vi "SELECT Template.vi"   [LabVIEW 2016]
uses:
  <vilib>/JDP Science/PostgreSQL Library/Result/PQ Result.lvclass
  <vilib>/JDP Science/PostgreSQL Library/Connection/PQ Connection.lvclass
  <vilib>/JDP Science/PostgreSQL Library/Connection/Execute Command (Result).vi
types:
  T1 = cluster{"Get:Get String":string, "Get:Get String":string, "Get:Get String":string, "Get:Get DBL":dbl}
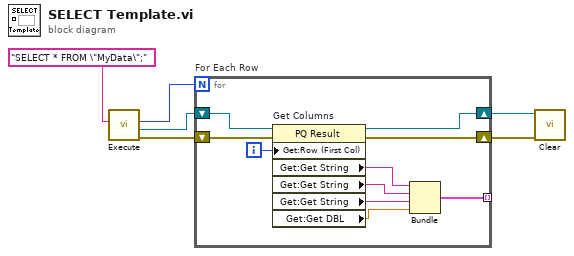
[diagram p0: block diagram]
diagram:
  n1 = call-poly <vilib>:"Execute.vi"("SQL"="SELECT * FROM \"MyData\";" ("command")) -> ("error out"=w4:errorcluster, "First Result with Rows returned"=w1:refnum<class "PQ Result.lvclass">, "Number of Rows"=w5:i32)  [unwired: 7 in, 1 out]
  n2 = for "For Each Row" {
    N: w5 -> [_]
    shift-right: [w16] -> w6
    shift-left: w1 -> [w9]
    shift-right: [w15] -> w3
    shift-left: w4 -> [w8]
    tunnel: [w10] -> _ mode=indexing
    i -> [w7]
    n3 = property on="Get Columns" class="PQ Result"(reference=w9, error in=w8, "Get:Row (First Col)"=w7) -> (reference out=w16:refnum<class "PQ Result.lvclass">, error out=w15:errorcluster, "Get:Get String"=w14:string, "Get:Get String"=w13:string, "Get:Get String"=w12:string, "Get:Get DBL"=w11:dbl)
    n4 = Bundle("Get:Get String"=w14, "Get:Get String"=w13, "Get:Get String"=w12, "Get:Get DBL"=w11) -> (w10:T1)  [unwired: 1 in]
  }
  n5 = call <vilib>:"Clear.vi"("error in (no error)"=w3, "PQ Result  in"=w6) -> ()  [unwired: 9 in, 1 out]
